vi "error_check.vi"(8 "error in (no error)":errorcluster, 10 "Response in":string) -> (0 "error out":errorcluster, 2 "Response out":string)   [LabVIEW 2018]
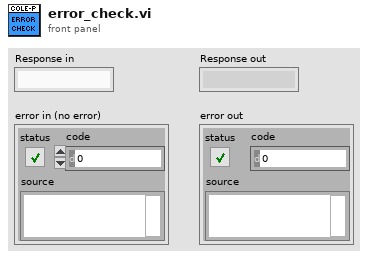
[diagram p1: front panel]
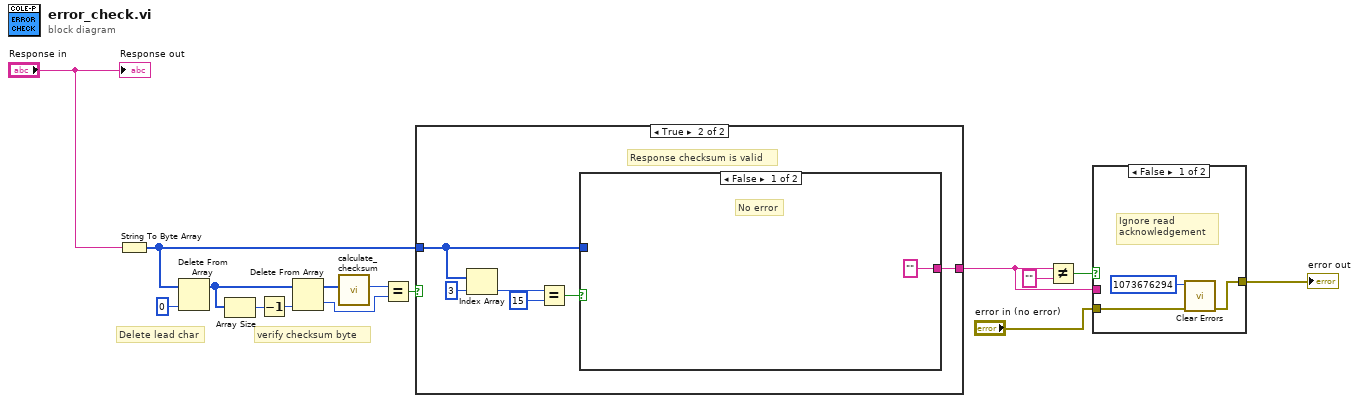
[diagram p0: block diagram]
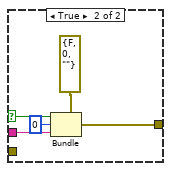
[diagram p2: hidden frame]
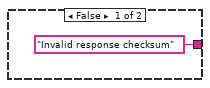
[diagram p3: hidden frame]
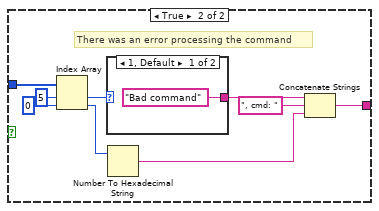
[diagram p4: hidden frame]
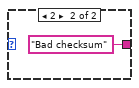
[diagram p5: hidden frame]
diagram:
  # "verify checksum byte"
  # "Delete lead char"
  n1 = String To Byte Array(string="Response in") -> (unsigned byte array=w2:u8[])
  n2 = Delete From Array(array=w2, index=0) -> (array with subset deleted=w8:u8[])  [unwired: 1 in, 1 out]
  n3 = Array Size(array=w8) -> (size(s)=w9:i32)
  n4 = Decrement(x=w9) -> (x-1=w10:i32)
  n5 = Delete From Array(array=w8, index=w10) -> (deleted portion=w6:u8, array with subset deleted=w4:u8[])  [unwired: 1 in]
  n6 = call "calculate_checksum.vi"("Byte array"=w4) -> ("Checksum"=w5:u8)  [unwired: 10 in]
  n7 = Equal?(x=w5, y=w6) -> (x = y?=w7:bool)
  n8 = case shown="True" w7 {
    tunnel: w2 -> [_ w18]
    tunnel: ["Invalid response checksum" w17] -> w14
    frame False {
    }
    frame True {
      # "Response checksum is valid"
      n9 = Index Array(array=w18, index=3) -> (element=w21:u8)
      n10 = Equal?(x=w21, y=u8 15) -> (x = y?=w19:bool)
      n11 = case shown="False" w19 {
        tunnel: w18 -> [_ w32]
        tunnel: ["" w24] -> w17
        frame False {
          # "No error"
        }
        frame True {
          # "There was an error processing the command"
          n12 = Index Array(array=w32, index #1=5 ("index"), index #2=0 ("index")) -> (element #1=w30:u8, element #2=w28:u8)
          n13 = case shown="1, Default" w30 {
            tunnel: ["Bad command" "Bad checksum"] -> w27
            frame 1, Default {
            }
            frame 2 {
            }
          }
          n14 = Number To Hexadecimal String(2:w28) -> (0:w25:string)  [unwired: 1 in]
          n15 = Concatenate Strings(w27, ", cmd: " ("string"), w25) -> (w24:string)
        }
      }
    }
  }
  n16 = Not Equal?(x=w14, y="") -> (x != y?=w12:bool)
  n17 = case shown="False" w12 {
    selector: w12 -> [_ w41]
    tunnel: [w36 w39] -> w15
    tunnel: "error in (no error)" -> [w37 _]
    tunnel: w14 -> [_ w40]
    frame False {
      # "Ignore read\nacknowledgement"
      n18 = call <vilib>:"Clear Errors.vi"("error in (no error)"=w37, "specific error code to clear (0: all)"=1073676294) -> ("error out"=w36:errorcluster)  [unwired: 4 in, 1 out]
    }
    frame True {
      n19 = Bundle(cluster=errorcluster {"status"=FALSE, "code"=0, "source"=""} ("error out"), "status"=w41, "code"=0, "source"=w40) -> (w39:errorcluster)
    }
  }
  "error out" <- w15
  "Response out" <- "Response in"
